vi "DB_test.vi"() -> ()   [LabVIEW 2019, in "Class 2.lvclass"]
uses:
  Class 2.lvclass
  <vilib>/addons/database/Connection.llb/DB Tools Open Connec (Path).vi
  <vilib>/addons/database/NI_Database_API.lvlib
panel:
  out "data":variant[][](array[variant])
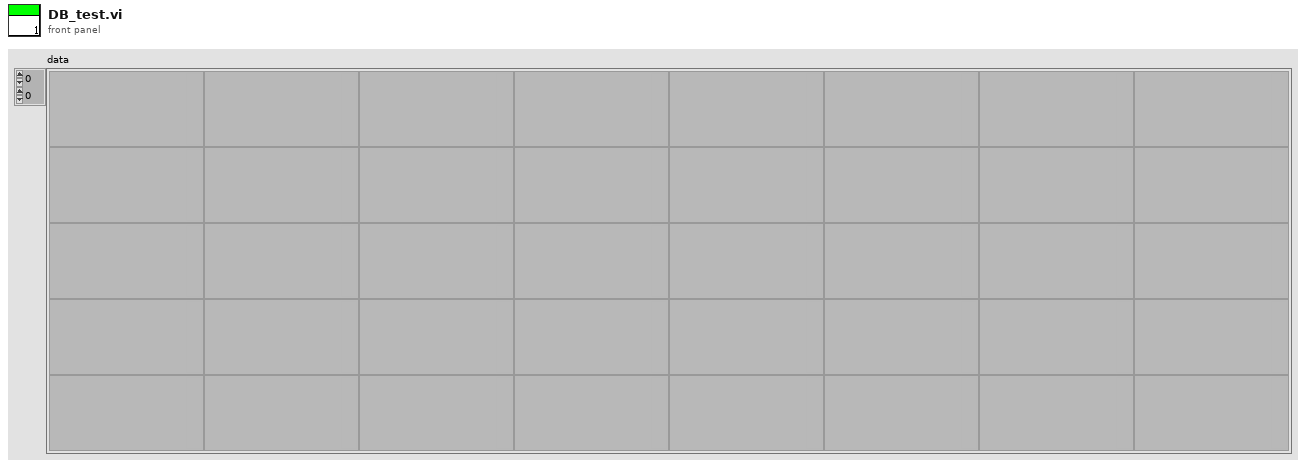
[diagram p1: front panel]
types:
  T1 = typedef "NI_Database_API.lvlib/Conn ObjectReference.ctl" = refnum<k1>
  T2 = cluster{"name or relative path":string, i8, i8, i8, i8, i8, i8}
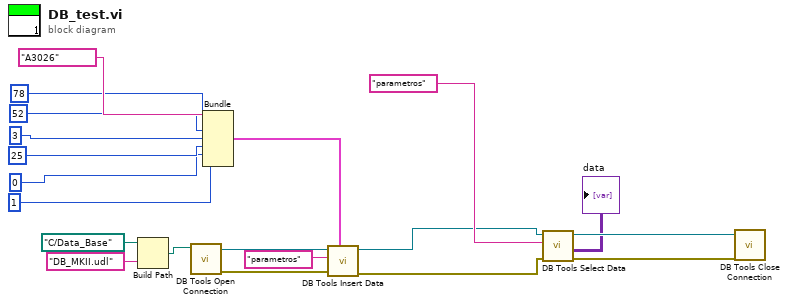
[diagram p0: block diagram]
diagram:
  n1 = Build Path(base path=path "C:/Data_Base", name or relative path="DB_MKII.udl") -> (appended path=w16:path)
  n2 = call-poly <vilib>:"DB Tools Open Connection.vi"("connection information"=w16) -> ("error out"=w13:errorcluster, "connection reference"=w14:T1)  [unwired: 7 in]
  n3 = Bundle("name or relative path"="A3026", i8 78, i8 52, i8 3, i8 25, i8 0, i8 1) -> (w9:T2)  [unwired: 1 in]
  n4 = call <vilib>:"DB Tools Insert Data.vi"("data"=w9, "error in (no error)"=w13, "table"="parametros", "connection reference"=w14) -> ("error out"=w10:errorcluster, "connection reference out"=w11:T1)  [unwired: 6 in]
  n5 = call <vilib>:"DB Tools Select Data.vi"("error in (no error)"=w10, "table"="parametros", "connection reference"=w11) -> ("error out"=w19:errorcluster, "data"=→"data":variant[][], "connection reference out"=w20:T1)  [unwired: 3 in]
  n6 = call <vilib>:"DB Tools Close Connection.vi"("error in (no error)"=w19, "connection reference"=w20) -> ()  [unwired: 5 in, 1 out]
